vi "SPI-BITBASH_read.vi"(10 "Read Address":u8, 11 "Mouse IO":T1={"SCK"="DIO18", "MISO"="DIO25", "MOSI"="DIO26", "CS"="DIO17"}) -> (2 "Data out":u8, 3 "Mouse IO Out":T1)   [LabVIEW 2012]
uses:
  <vilib>/rvi/eio/common/nirviEmuTemplateMethod_errors.vi
  <vilib>/eio/EIONode/EIONode.xnode
panel:
  out "Array":bool[](array[boolean])
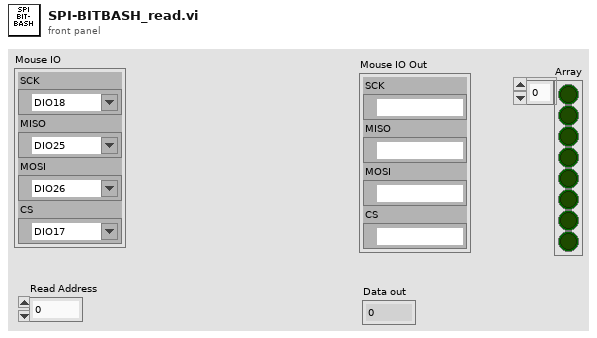
[diagram p1: front panel]
types:
  T1 = cluster{"SCK":refnum<k21>, "MISO":refnum<k21>, "MOSI":refnum<k21>, "CS":refnum<k21>}
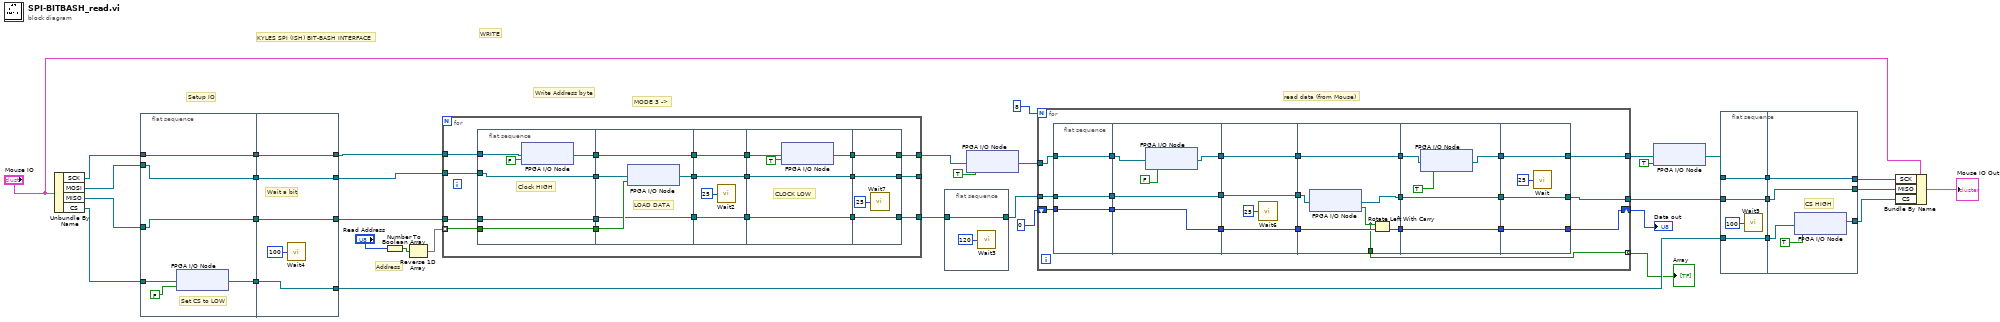
[diagram p0: block diagram]
diagram:
  # "MODE 3 ->"
  # "Setup IO"
  # "KYLES SPI (ISH) BIT-BASH INTERFACE"
  # "WRITE"
  # "read data (from Mouse)"
  # "Write Address byte"
  # "Address"
  n1 = Unbundle By Name("Mouse IO") -> ("SCK"=w20:refnum<k21>, "MOSI"=w19:refnum<k21>, "MISO"=w12:refnum<k21>, "CS"=w18:refnum<k21>)
  n2 = flat-sequence {
    tunnel: [w41] -> w32
    tunnel: w20 -> [w39]
    tunnel: w19 -> [w38]
    tunnel: w18 -> [w40]
    tunnel: [w39] -> w17
    tunnel: [w38] -> w15
    tunnel: w12 -> [w37]
    tunnel: [w37] -> w11
    tunnel: [w46] -> w29
    tunnel: w32 -> [w46]
    tunnel: [w45] -> w16
    tunnel: w17 -> [w45]
    tunnel: [w44] -> w14
    tunnel: w15 -> [w44]
    tunnel: [w43] -> w10
    tunnel: w11 -> [w43]
    frame #0 {
      # "Set CS to LOW"
      n3 = xnode "FPGA I/O Node"("I/O Item"=FALSE, "FPGA I/O In"=w40) -> ("FPGA I/O Out"=w41:refnum<k21>)
    }
    frame #1 {
      # "Wait a bit"
      n4 = call "Wait4"("Count(uSec)"=u32 100) -> ()  [unwired: 1 out]
    }
  }
  n5 = Number To Boolean Array(number="Read Address") -> (Boolean array=w33:bool[])
  n6 = Reverse 1D Array(array=w33) -> (reversed array=w13:bool[])
  n7 = for {
    tunnel: w13 -> [w67] mode=indexing
    tunnel: [w66] -> w34
    tunnel: [w65] -> _
    tunnel: w16 -> [w60]
    tunnel: w14 -> [w59]
    tunnel: w10 -> [w56]
    tunnel: [w54] -> w4
    n8 = flat-sequence {
      tunnel: [w72] -> w62
      tunnel: [w71] -> w61
      tunnel: w67 -> [w71]
      tunnel: w60 -> [w70]
      tunnel: w59 -> [w69]
      tunnel: [w69] -> w58
      tunnel: [w68] -> w57
      tunnel: w56 -> [w68]
      tunnel: [w78] -> w51
      tunnel: [w77] -> w53
      tunnel: [w74] -> w49
      tunnel: w57 -> [w74]
      tunnel: w58 -> [w75]
      tunnel: w61 -> [w76]
      tunnel: w62 -> [w78]
      tunnel: w53 -> [w82]
      tunnel: [w82] -> w52
      tunnel: w51 -> [w81]
      tunnel: [w81] -> w50
      tunnel: w49 -> [w80]
      tunnel: [w80] -> w48
      tunnel: [w85] -> w64
      tunnel: [w84] -> w63
      tunnel: w52 -> [w84]
      tunnel: w50 -> [w86]
      tunnel: [w83] -> w55
      tunnel: w48 -> [w83]
      tunnel: [w89] -> w65
      tunnel: [w91] -> w66
      tunnel: w64 -> [w91]
      tunnel: w63 -> [w89]
      tunnel: w55 -> [w90]
      tunnel: [w90] -> w54
      frame #0 {
        # "Clock HIGH"
        n9 = xnode "FPGA I/O Node"("I/O Item"=FALSE, "FPGA I/O In"=w70) -> ("FPGA I/O Out"=w72:refnum<k21>)
      }
      frame #1 {
        # "LOAD DATA"
        n10 = xnode "FPGA I/O Node"("I/O Item"=w76, "FPGA I/O In"=w75) -> ("FPGA I/O Out"=w77:refnum<k21>)
      }
      frame #2 {
        n11 = call "Wait2"("Count(uSec)"=u16 25) -> ()  [unwired: 1 out]
      }
      frame #3 {
        # "CLOCK LOW"
        n12 = xnode "FPGA I/O Node"("I/O Item"=TRUE, "FPGA I/O In"=w86) -> ("FPGA I/O Out"=w85:refnum<k21>)
      }
      frame #4 {
        n13 = call "Wait7"("Count(uSec)"=u16 25) -> ()  [unwired: 1 out]
      }
    }
  }
  n14 = flat-sequence {
    tunnel: w4 -> [w93]
    tunnel: [w93] -> w3
    frame #0 {
      n15 = call "Wait3"("Count(uSec)"=u32 120) -> ()  [unwired: 1 out]
    }
  }
  n16 = xnode "FPGA I/O Node"("I/O Item"=TRUE, "FPGA I/O In"=w34) -> ("FPGA I/O Out"=w25:refnum<k21>)
  n17 = for {
    N: 8 -> [_]
    tunnel: w25 -> [w96]
    tunnel: [w115] -> w31
    tunnel: w3 -> [w112]
    tunnel: [w111] -> w8
    shift-right: [w108] -> w5
    shift-left: u8 0 -> [w110]
    tunnel: [w94] -> w2 mode=indexing
    n18 = flat-sequence {
      tunnel: [w116] -> w114
      tunnel: [w118] -> w113
      tunnel: [w117] -> w109
      tunnel: w112 -> [w118]
      tunnel: w110 -> [w117]
      tunnel: w96 -> [w116]
      tunnel: w114 -> [w122]
      tunnel: [w121] -> w107
      tunnel: w113 -> [w120]
      tunnel: [w120] -> w105
      tunnel: w109 -> [w119]
      tunnel: [w119] -> w103
      tunnel: w107 -> [w127]
      tunnel: [w127] -> w106
      tunnel: w105 -> [w126]
      tunnel: [w126] -> w104
      tunnel: w103 -> [w125]
      tunnel: [w125] -> w102
      tunnel: w106 -> [w133]
      tunnel: w104 -> [w132]
      tunnel: w102 -> [w130]
      tunnel: [w133] -> w101
      tunnel: [w131] -> w100
      tunnel: [w129] -> w99
      tunnel: [w128] -> w94
      tunnel: w101 -> [w134]
      tunnel: w100 -> [w138]
      tunnel: w99 -> [w137]
      tunnel: [w138] -> w98
      tunnel: [w137] -> w97
      tunnel: [w135] -> w95
      tunnel: [w140] -> w108
      tunnel: [w141] -> w111
      tunnel: [w142] -> w115
      tunnel: w98 -> [w141]
      tunnel: w97 -> [w140]
      tunnel: w95 -> [w142]
      frame #0 {
      }
      frame #1 {
        n19 = xnode "FPGA I/O Node"("I/O Item"=FALSE, "FPGA I/O In"=w122) -> ("FPGA I/O Out"=w121:refnum<k21>)
      }
      frame #2 {
        n20 = call "Wait6"("Count(uSec)"=u16 25) -> ()  [unwired: 1 out]
      }
      frame #3 {
        n21 = xnode "FPGA I/O Node"("FPGA I/O In"=w132) -> ("I/O Item"=w128:bool, "FPGA I/O Out"=w131:refnum<k21>)
        n22 = Rotate Left With Carry(2:w130, 3:w128) -> (0:w129:u8)  [unwired: 1 out]
      }
      frame #4 {
        n23 = xnode "FPGA I/O Node"("I/O Item"=TRUE, "FPGA I/O In"=w134) -> ("FPGA I/O Out"=w135:refnum<k21>)
      }
      frame #5 {
        n24 = call "Wait"("Count(uSec)"=u16 25) -> ()  [unwired: 1 out]
      }
    }
  }
  "Data out" <- w5
  "Array" <- w2
  n25 = xnode "FPGA I/O Node"("I/O Item"=TRUE, "FPGA I/O In"=w31) -> ("FPGA I/O Out"=w23:refnum<k21>)
  n26 = flat-sequence {
    tunnel: w29 -> [w145]
    tunnel: w23 -> [w146]
    tunnel: [w146] -> w27
    tunnel: [w145] -> w26
    tunnel: [w143] -> w9
    tunnel: w8 -> [w143]
    tunnel: [w151] -> w30
    tunnel: [w148] -> w28
    tunnel: w27 -> [w151]
    tunnel: w26 -> [w150]
    tunnel: w9 -> [w147]
    tunnel: [w147] -> w7
    frame #0 {
      n27 = call "Wait5"("Count(uSec)"=u32 100) -> ()  [unwired: 1 out]
    }
    frame #1 {
      # "CS HIGH"
      n28 = xnode "FPGA I/O Node"("I/O Item"=TRUE, "FPGA I/O In"=w150) -> ("FPGA I/O Out"=w148:refnum<k21>)
    }
  }
  n29 = Bundle By Name(cluster="Mouse IO", "SCK"=w30, "MISO"=w7, "CS"=w28) -> (→"Mouse IO Out":T1)
